vi "FlatToRichcif_manager_PluginStatus.vi"(5 "OutputClusterType":T1, 11 "InputCluster":T12) -> (3 "OutputCluster":T1)   [LabVIEW 2021, in "CIF_Manager_server.lvlib"]
uses:
  CIF_Manager_server.lvlib
  cif_manager_PluginStatus_Flat.ctl
  cif_manager_PluginName_Flat.ctl
  cif_plugincore_StatusData_Flat.ctl
  cif_plugincore_StatusData_State.ctl
  cif_plugincore_TimingStatistics_Flat.ctl
  cif_common_TimingStats_Flat.ctl
  cif_plugincore_FifoStatistics_Flat.ctl
  cif_plugincore_Error_Flat.ctl
  cif_plugincore_MonitorDoubles_Flat.ctl
  cif_plugincore_MonitorU64_Flat.ctl
  cif_plugincore_MonitorI64_Flat.ctl
  cif_manager_PluginStatus.ctl
  cif_manager_PluginName.ctl
  cif_plugincore_StatusData.ctl
  cif_plugincore_TimingStatistics.ctl
  cif_common_TimingStats.ctl
  cif_plugincore_FifoStatistics.ctl
  cif_plugincore_Error.ctl
  cif_plugincore_MonitorDoubles.ctl
  cif_plugincore_MonitorU64.ctl
  cif_plugincore_MonitorI64.ctl
  FlatToRichcif_plugincore_TimingStatistics.vi
  FlatToRichcif_plugincore_FifoStatistics.vi
  FlatToRichcif_plugincore_Error.vi
  FlatToRichcif_plugincore_MonitorDoubles.vi
  FlatToRichcif_plugincore_MonitorU64.vi
  FlatToRichcif_plugincore_MonitorI64.vi
  FlatToRichcif_common_TimingStats.vi
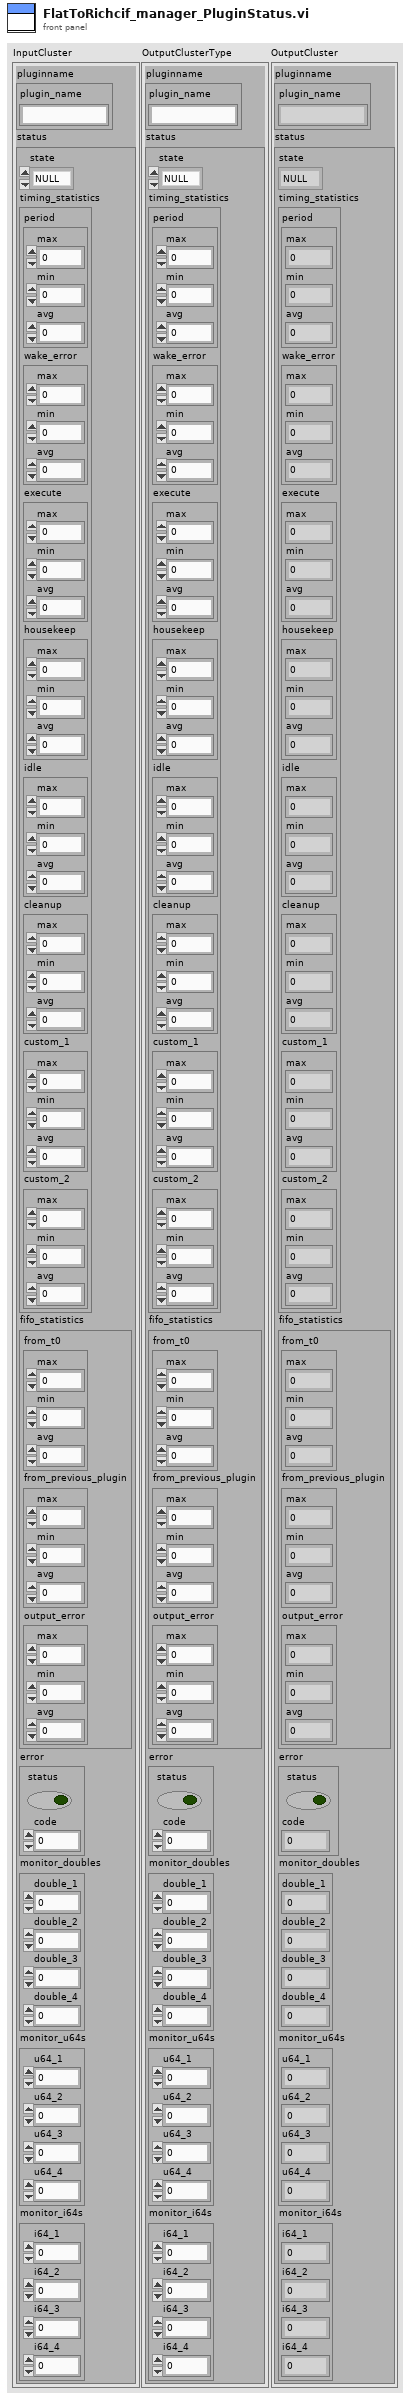
[diagram p1: front panel]
types:
  T1 = typedef "CIF_Manager_server.lvlib/cif_manager_PluginStatus.ctl" = cluster{"pluginname":T2, "status":T3}
  T2 = typedef "CIF_Manager_server.lvlib/cif_manager_PluginName.ctl" = cluster{"plugin_name":string}
  T3 = typedef "CIF_Manager_server.lvlib/cif_plugincore_StatusData.ctl" = cluster{"state":T4, "timing_statistics":T5, "fifo_statistics":T7, "error":T8, "monitor_doubles":T9, "monitor_u64s":T10, "monitor_i64s":T11}
  T4 = typedef "CIF_Manager_server.lvlib/cif_plugincore_StatusData_State.ctl" = enum32{"NULL", "CREATING", "LISTENING", "RUNNING", "CLEANINGUP", "DESTROYING"}
  T5 = typedef "CIF_Manager_server.lvlib/cif_plugincore_TimingStatistics.ctl" = cluster{"period":T6, "wake_error":T6, "execute":T6, "housekeep":T6, "idle":T6, "cleanup":T6, "custom_1":T6, "custom_2":T6}
  T6 = typedef "CIF_Manager_server.lvlib/cif_common_TimingStats.ctl" = cluster{"max":i64, "min":i64, "avg":dbl}
  T7 = typedef "CIF_Manager_server.lvlib/cif_plugincore_FifoStatistics.ctl" = cluster{"from_t0":T6, "from_previous_plugin":T6, "output_error":T6}
  T8 = typedef "CIF_Manager_server.lvlib/cif_plugincore_Error.ctl" = cluster{"status":bool, "code":i32}
  T9 = typedef "CIF_Manager_server.lvlib/cif_plugincore_MonitorDoubles.ctl" = cluster{"double_1":dbl, "double_2":dbl, "double_3":dbl, "double_4":dbl}
  T10 = typedef "CIF_Manager_server.lvlib/cif_plugincore_MonitorU64.ctl" = cluster{"u64_1":u64, "u64_2":u64, "u64_3":u64, "u64_4":u64}
  T11 = typedef "CIF_Manager_server.lvlib/cif_plugincore_MonitorI64.ctl" = cluster{"i64_1":i64, "i64_2":i64, "i64_3":i64, "i64_4":i64}
  T12 = typedef "CIF_Manager_server.lvlib/cif_manager_PluginStatus_Flat.ctl" = cluster{"pluginname":T13, "status":T14}
  T13 = typedef "CIF_Manager_server.lvlib/cif_manager_PluginName_Flat.ctl" = cluster{"plugin_name":string}
  T14 = typedef "CIF_Manager_server.lvlib/cif_plugincore_StatusData_Flat.ctl" = cluster{"state":T4, "timing_statistics":T15, "fifo_statistics":T17, "error":T18, "monitor_doubles":T19, "monitor_u64s":T20, "monitor_i64s":T21}
  T15 = typedef "CIF_Manager_server.lvlib/cif_plugincore_TimingStatistics_Flat.ctl" = cluster{"period":T16, "wake_error":T16, "execute":T16, "housekeep":T16, "idle":T16, "cleanup":T16, "custom_1":T16, "custom_2":T16}
  T16 = typedef "CIF_Manager_server.lvlib/cif_common_TimingStats_Flat.ctl" = cluster{"max":i64, "min":i64, "avg":dbl}
  T17 = typedef "CIF_Manager_server.lvlib/cif_plugincore_FifoStatistics_Flat.ctl" = cluster{"from_t0":T16, "from_previous_plugin":T16, "output_error":T16}
  T18 = typedef "CIF_Manager_server.lvlib/cif_plugincore_Error_Flat.ctl" = cluster{"status":bool, "code":i32}
  T19 = typedef "CIF_Manager_server.lvlib/cif_plugincore_MonitorDoubles_Flat.ctl" = cluster{"double_1":dbl, "double_2":dbl, "double_3":dbl, "double_4":dbl}
  T20 = typedef "CIF_Manager_server.lvlib/cif_plugincore_MonitorU64_Flat.ctl" = cluster{"u64_1":u64, "u64_2":u64, "u64_3":u64, "u64_4":u64}
  T21 = typedef "CIF_Manager_server.lvlib/cif_plugincore_MonitorI64_Flat.ctl" = cluster{"i64_1":i64, "i64_2":i64, "i64_3":i64, "i64_4":i64}
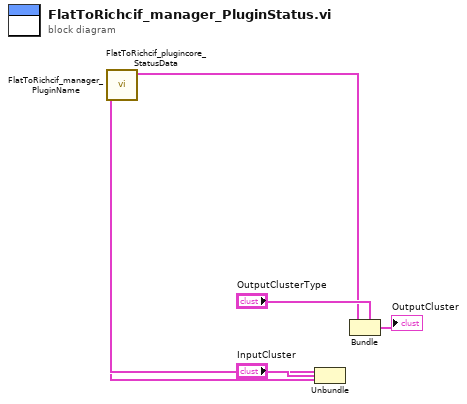
[diagram p0: block diagram]
diagram:
  n1 = Unbundle "Unbundle"("InputCluster") -> ("pluginname"=w4:T13, "status"=w2:T14)
  n2 = call "FlatToRichcif_plugincore_StatusData.vi"("InputCluster"=w2) -> ("OutputCluster"=w1:T3)  [unwired: 10 in]
  n3 = call "FlatToRichcif_manager_PluginName.vi"("InputCluster"=w4) -> ("OutputCluster"=w3:T2)  [unwired: 10 in]
  n4 = Bundle "Bundle"(cluster="OutputClusterType", "pluginname"=w3, "status"=w1) -> (→"OutputCluster":T1)
